vi "Solve influence matrix equation.vi"(0 "Triangle panels in":T1[](array[typedef]), 1 "U_inf":sgl[](array[numeric])=[1.0, 0.0, 0.0], 2 "res. tol.":dbl=9.99999993922529e-09, 3 "max. iters":i32=100, 4 "solver method":u8(ring) items=["Jacobi (rel.)", "Jacobi (abs.)", "Gauss-Seidel (rel.)", "Gauss-Seidel (abs.)", "NI solver"]) -> (6 "sys. residual":sgl, 7 "Triangle panels out":T1[](array[typedef]), 8 "G'":sgl[](array[numeric])=[1.0, 2.0, -1.0, 1.0], 9 "Iterations":i32=10, 10 "Converged?":bool=TRUE)   [LabVIEW 2017]
uses:
  ctls/Triangle panel.ctl
  <vilib>/Analysis/7linalg.llb/Solve Linear Equations (single right hand).vi
  <vilib>/Analysis/baseanly.llb/A x Vector.vi
  <vilib>/Analysis/baseanly.llb/Solve Linear Equations By Cholesky.vi
  <vilib>/Analysis/baseanly.llb/Real Matrix to Compact Array.vi
  <vilib>/Analysis/baseanly.llb/Real Compact Tri-Matrix Linear Eqs.vi
  Biot-Savart induced velocity.vi
  <vilib>/Analysis/7linalg.llb/Solve Linear Eqs (General).vi
  <vilib>/Analysis/7linalg.llb/Solve Linear Eqs (Gen, single right hand).vi
  <vilib>/Analysis/NI_AALPro.lvlib
  <vilib>/Analysis/NI_AALBase.lvlib
panel:
  out "i":i32(graph)
  # "PN 22/10/17"
  # "Vertices"
  # "Edges"
  # "Unit normal"
  # "Control point"
  # "Edge\nlinks \n(tri index)"
  # "Vertices"
  # "Edges"
  # "Unit normal"
  # "Control point"
  # "Edge\nlinks \n(tri index)"
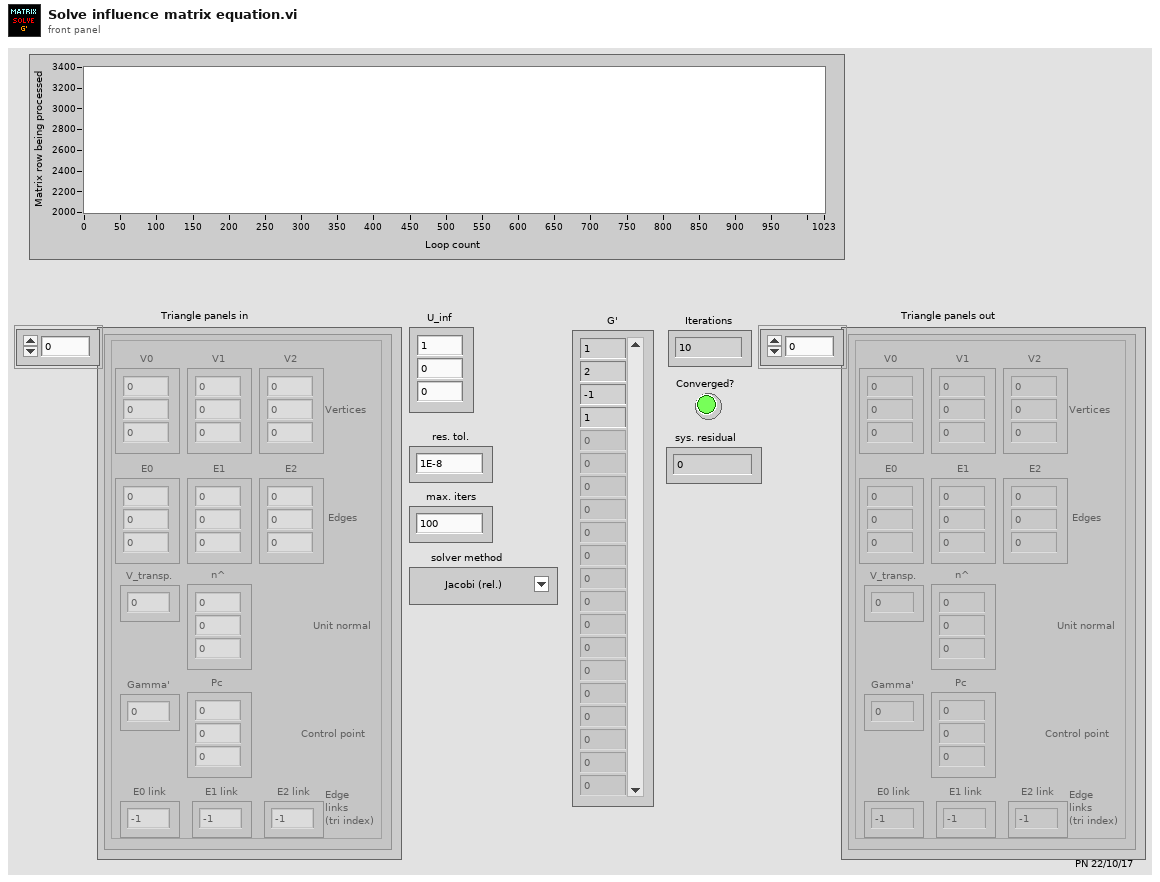
[diagram p1: front panel]
types:
  T1 = typedef "Triangle panel.ctl" = cluster{"V0":sgl[], "V1":sgl[], "V2":sgl[], "E0":sgl[], "E1":sgl[], "E2":sgl[], "n^":sgl[], "Pc":sgl[], "Gamma'":sgl, "V_transp.":sgl, "E0 link":i32, "E1 link":i32, "E2 link":i32}
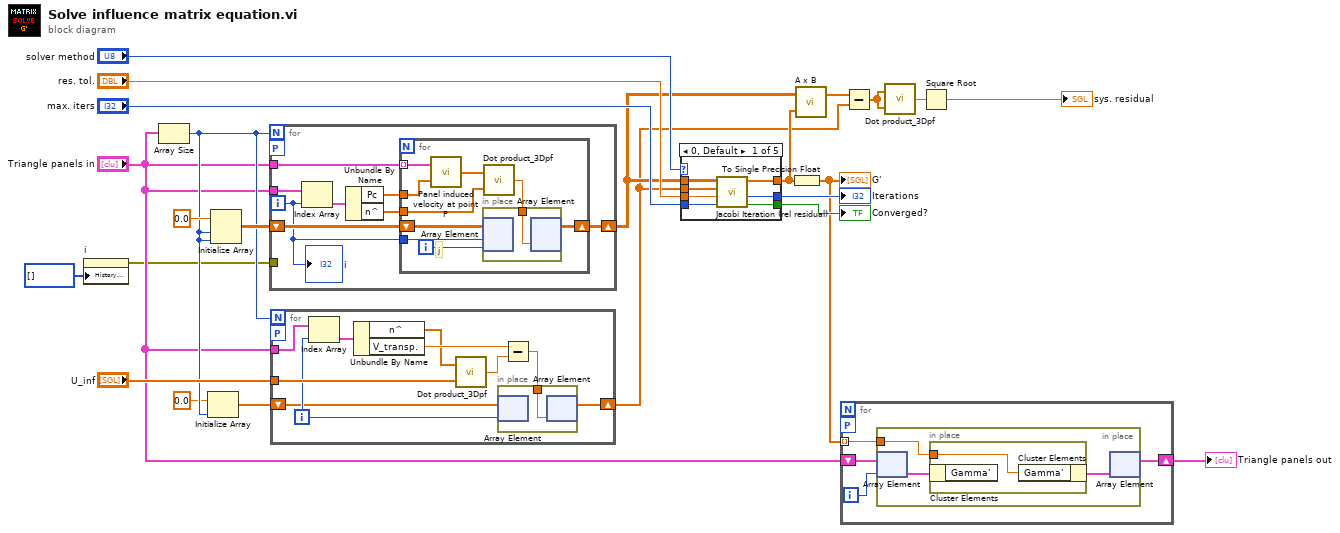
[diagram p0: block diagram]
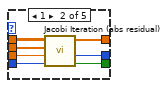
[diagram p2: hidden frame]
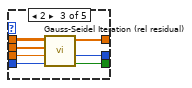
[diagram p3: hidden frame]
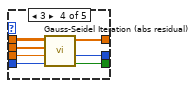
[diagram p4: hidden frame]
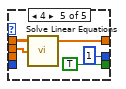
[diagram p5: hidden frame]
diagram:
  n1 = property on="i" class="WFChart (strict)"("History Data"=i32[] []) -> (error out=w1:errorcluster)  [unwired: 2 in, 1 out]
  n2 = Array Size(array="Triangle panels in") -> (size(s)=w7:i32)
  n3 = Initialize Array(sgl 0.0 ("element"), w7) -> (w5:sgl[])
  n4 = Initialize Array(sgl 0.0 ("element"), w7, w7) -> (w10:sgl[][])
  n5 = for {
    N: w7 -> [_]
    tunnel: "Triangle panels in" -> [w31]
    workers-P: _ -> [_]
    shift-right: [w26] -> w9
    shift-left: w10 -> [w27]
    tunnel: "Triangle panels in" -> [w25]
    tunnel: w1 -> [_]
    i -> [w24]
    n6 = Index Array(array=w25, index=w24) -> (element=w30:T1)
    n7 = Unbundle By Name(w30) -> ("Pc"=w29:sgl[], "n^"=w28:sgl[])
    n8 = for {
      tunnel: w31 -> [w40] mode=indexing
      tunnel: w29 -> [w39]
      tunnel: w28 -> [w38]
      shift-right: [w35] -> w26
      shift-left: w27 -> [w36]
      tunnel: w24 -> [w33]
      i -> [w32]
      # "j"
      n9 = call "Panel induced velocity at point P.vi"("P"=w39, "Triangle panel"=w40) -> ("U / G'"=w37:sgl[])
      n10 = call "Dot product_3Dpf.vi"("B"=w38, "A"=w37) -> ("A . B"=w34:sgl)
      n11 = in-place {
        in-place-border: w34 -> [w41]
        n12 = in-place-array #1(w36, w33, w32) -> ()  [unwired: 1 out]
        n13 = in-place-array #1(w41) -> (w35:sgl[][])  [unwired: 2 out]
      }
    }
    "i" <- w24
  }
  n14 = for {
    N: w7 -> [_]
    tunnel: "Triangle panels in" -> [w51]
    tunnel: "U_inf" -> [w47]
    workers-P: _ -> [_]
    shift-right: [w43] -> w4
    shift-left: w5 -> [w42]
    i -> [w45]
    n15 = Index Array(array=w51, index=w45) -> (element=w50:T1)
    n16 = Unbundle By Name(w50) -> ("n^"=w48:sgl[], "V_transp."=w49:sgl)
    n17 = call "Dot product_3Dpf.vi"("B"=w47, "A"=w48) -> ("A . B"=w46:sgl)
    n18 = Subtract(x=w49, y=w46) -> (x-y=w44:sgl)
    n19 = in-place {
      in-place-border: w44 -> [w52]
      n20 = in-place-array #2(w42, w45) -> ()  [unwired: 1 out]
      n21 = in-place-array #2(w52) -> (w43:sgl[])  [unwired: 1 out]
    }
  }
  n22 = case shown="0, Default" "solver method" {
    tunnel: w9 -> [w59 w62 w73 w80 w85]
    tunnel: w4 -> [w58 w61 w72 w79 w84]
    tunnel: "res. tol." -> [w57 w60 w71 w78 _]
    tunnel: "max. iters" -> [w56 w66 w70 w77 _]
    tunnel: [w55 w64 w68 w74 TRUE ("Converged?")] -> w21
    tunnel: [w54 w65 w67 w75 1 ("Iterations")] -> w20
    tunnel: [w53 w63 w69 w76 w83] -> w17
    frame 0, Default {
      n23 = call "Jacobi Iteration (rel residual).vi"("max. iters"=w56, "res. tol"=w57, "B"=w58, "A"=w59) -> ("Converged?"=w55:bool, "Iterations"=w54:i32, "X"=w53:dbl[])  [unwired: 1 in]
    }
    frame 1 {
      n24 = call "Jacobi Iteration (abs residual).vi"("max. iters"=w66, "abs. tol"=w60, "B"=w61, "A"=w62) -> ("Converged?"=w64:bool, "Iterations"=w65:i32, "X"=w63:dbl[])  [unwired: 1 in]
    }
    frame 2 {
      n25 = call "Gauss-Seidel Iteration (rel residual).vi"("max. iters"=w70, "res. tol"=w71, "B"=w72, "A"=w73) -> ("Converged?"=w68:bool, "Iterations"=w67:i32, "X"=w69:dbl[])  [unwired: 1 in]
    }
    frame 3 {
      n26 = call "Gauss-Seidel Iteration (abs residual).vi"("max. iters"=w77, "res. tol"=w78, "B"=w79, "A"=w80) -> ("Converged?"=w74:bool, "Iterations"=w75:i32, "X"=w76:dbl[])  [unwired: 1 in]
    }
    frame 4 {
      n27 = call-poly <vilib>:"Solve Linear Equations.vi"("Known Vector"=w84, "Input Matrix"=w85) -> ("Solution Vector"=w83:dbl[])  [unwired: 1 in, 1 out]
    }
  }
  "Converged?" <- w21
  "Iterations" <- w20
  n28 = To Single Precision Float(number=w17) -> (single precision float=w18:sgl[])
  "G'" <- w18
  n29 = call-poly <vilib>:"A x B.vi"("Vector"=w17, "A"=w9) -> ("A x Vector"=w16:dbl[])  [unwired: 1 out]
  n30 = for {
    tunnel: w18 -> [w89] mode=indexing
    workers-P: _ -> [_]
    shift-right: [w86] -> w8
    shift-left: "Triangle panels in" -> [w88]
    i -> [w87]
    n31 = in-place {
      in-place-border: w89 -> [w92]
      n32 = in-place-array #3(w88, w87) -> (w91:T1)
      n33 = in-place {
        in-place-border: w92 -> [w93]
        n34 = in-place-cluster #4(w91) -> ()  [unwired: 1 out]
        n35 = in-place-cluster #4("Gamma'"=w93) -> (w90:T1)
      }
      n36 = in-place-array #3(w90) -> (w86:T1[])  [unwired: 1 out]
    }
  }
  "Triangle panels out" <- w8
  n37 = Subtract(x=w16, y=w4) -> (x-y=w15:dbl[])
  n38 = call "Dot product_3Dpf.vi"("B"=w15, "A"=w15) -> ("A . B"=w14:sgl)
  n39 = Square Root(x=w14) -> (sqrt(x)=→"sys. residual":sgl)
